vi "NB_SetProperty.vi"(0 "object in":refnum<class "NativeBaseTemplate.lvclass">, 1 "Property":bool, 5 "Error In":errorcluster) -> (14 "object out":refnum<class "NativeBaseTemplate.lvclass">, 19 "Error Out":errorcluster)   [LabVIEW 2020, in "NativeBaseTemplate.lvclass"]
uses:
  NativeBaseTemplate.lvclass
  NativeBaseTemplate.lvclass/NativeBaseTemplate.ctl
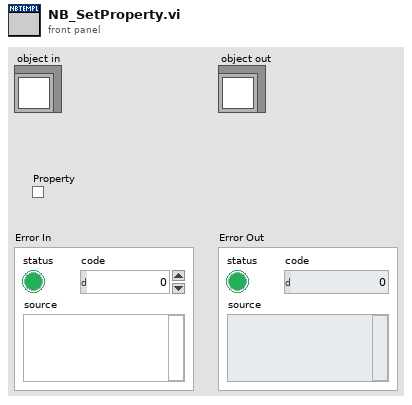
[diagram p1: front panel]
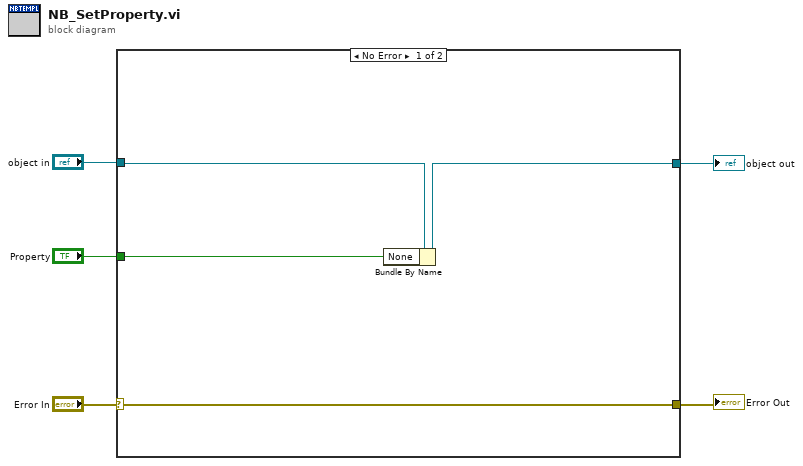
[diagram p0: block diagram]
diagram:
  n1 = case shown="No Error" "Error In" {
    selector: "Error In" -> [w8 w11]
    tunnel: [w8 w11] -> w4
    tunnel: [w6 w10] -> w2
    tunnel: "object in" -> [w7 w10]
    tunnel: "Property" -> [w9 _]
    frame No Error {
      n2 = Bundle By Name(cluster=w7, "None"=w9) -> (w6:refnum<class "NativeBaseTemplate.lvclass">)
    }
    frame Error {
    }
  }
  "Error Out" <- w4
  "object out" <- w2
